vi "Voltage Channels Array.vi"(0 "Channel 1":string, 5 "Relays Array In":bool[](array[boolean])=[FALSE, FALSE, FALSE, FALSE, FALSE, FALSE, FALSE, FALSE, FALSE, FALSE, FALSE, FALSE, FALSE, FALSE, FALSE, FALSE, FALSE, FALSE, FALSE, FALSE, FALSE, FALSE, FALSE, FALSE, FALSE, FALSE, FALSE, FALSE, FALSE, FALSE, FALSE, FALSE, FALSE, FALSE, FALSE, FALSE, FALSE, FALSE, FALSE, FALSE, FALSE, FALSE, FALSE, FALSE, FALSE, FALSE, FALSE, FALSE, FALSE, FALSE, FALSE, FALSE, FALSE, FALSE, FALSE, FALSE, FALSE, FALSE, FALSE, FALSE, FALSE, FALSE, FALSE, FALSE, FALSE, FALSE, FALSE, FALSE, FALSE, FALSE, FALSE, FALSE, FALSE, FALSE, FALSE, FALSE, FALSE, FALSE, FALSE, FALSE, FALSE, FALSE, FALSE, FALSE, FALSE, FALSE, FALSE, FALSE, FALSE, FALSE, FALSE, FALSE, FALSE, FALSE, FALSE, FALSE], 11 "error in":errorcluster, 13 "State":bool) -> (6 "Relay Array out":bool[](array[boolean]), 15 "error out":errorcluster)   [LabVIEW 2021, in "DMM_Scan DAQ Ext RLY.lvlib"]
doc: "Change the Relay Array State to Open/Close the corresponding multiplexer channels for Voltage Type Relays."
uses:
  DMM_Scan DAQ Ext RLY.lvlib
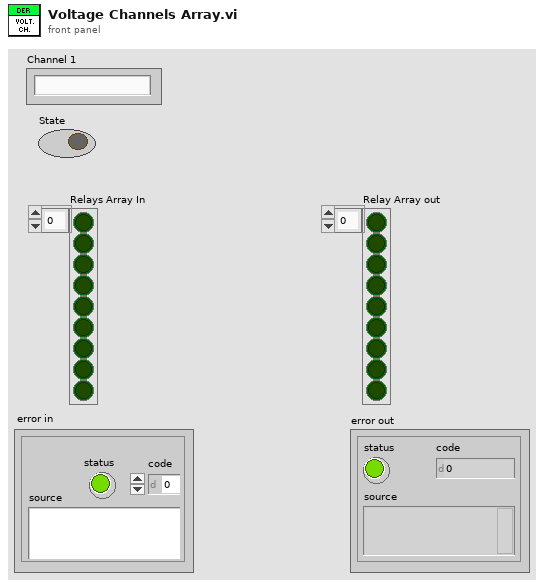
[diagram p1: front panel]
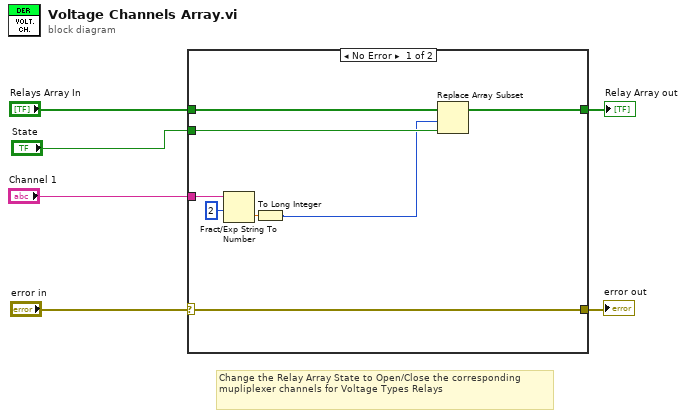
[diagram p0: block diagram]
diagram:
  # "Change the Relay Array State to Open/Close the corresponding mupliplexer channels for Voltage Types Relays"
  n1 = case shown="No Error" "error in" {
    selector: "error in" -> [w12 w16]
    tunnel: "Channel 1" -> [w11 _]
    tunnel: [w12 w16] -> w4
    tunnel: "Relays Array In" -> [w9 w15]
    tunnel: [w10 w15] -> w2
    tunnel: "State" -> [w8 _]
    frame No Error {
      n2 = Fract/Exp String To Number(string=w11, offset=2 ("offset (0)")) -> (number=w13:dbl)  [unwired: 2 in, 1 out]
      n3 = To Long Integer(number=w13) -> (32bit integer=w7:i32)
      n4 = Replace Array Subset(array=w9, new element=w8, index=w7) -> (w10:bool[])
    }
    frame Error {
    }
  }
  "error out" <- w4
  "Relay Array out" <- w2
